vi "Deadzone (SubVI).vi"(8 "Input":dbl, 11 "Deadzone":dbl) -> (0 "Input 2":dbl)   [LabVIEW 2020]
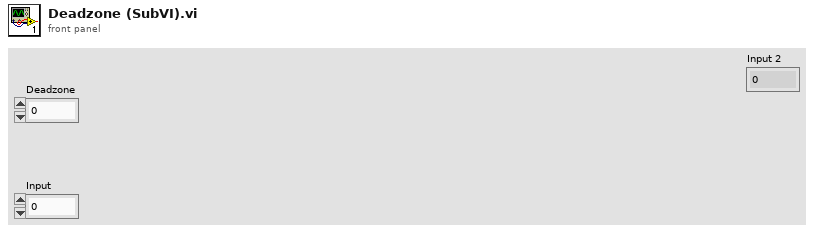
[diagram p1: front panel]
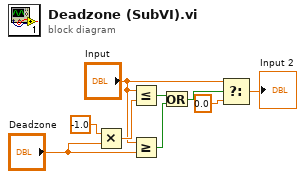
[diagram p0: block diagram]
diagram:
  n1 = Multiply(x=-1.0, y="Deadzone") -> (x*y=w6:dbl)
  n2 = Less Or Equal?(x="Input", y=w6) -> (x <= y?=w5:bool)
  n3 = Greater Or Equal?(x="Input", y="Deadzone") -> (x >= y?=w9:bool)
  n4 = Or(x=w5, y=w9) -> (x .or. y?=w4:bool)
  n5 = Select(t="Input", s=w4, f=0.0) -> (s? t:f=→"Input 2":dbl)
